vi "ParseAquatrakRange.vi"(8 "error in":errorcluster, 11 "Incoming String":string) -> (0 "error out":errorcluster, 1 "Cal Counts":i32, 2 "Valid Data":bool, 3 "Range":dbl, 5 "Range Counts":i32)   [LabVIEW 2019, in "Acquisition.lvlib"]
doc: "This VI takes an incoming string from the 4100 model Aquatrak controller and then outputs the quality as a Good Data = true/false boolean indicator."
uses:
  Acquisition/Acquisition.lvlib
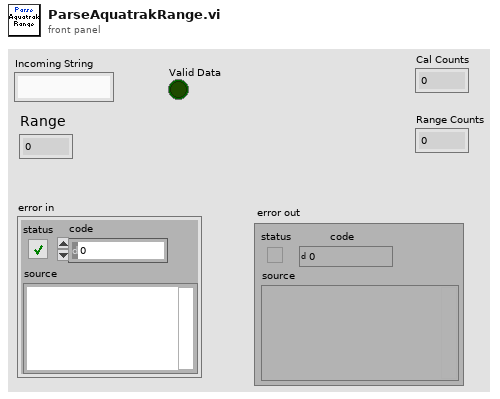
[diagram p1: front panel]
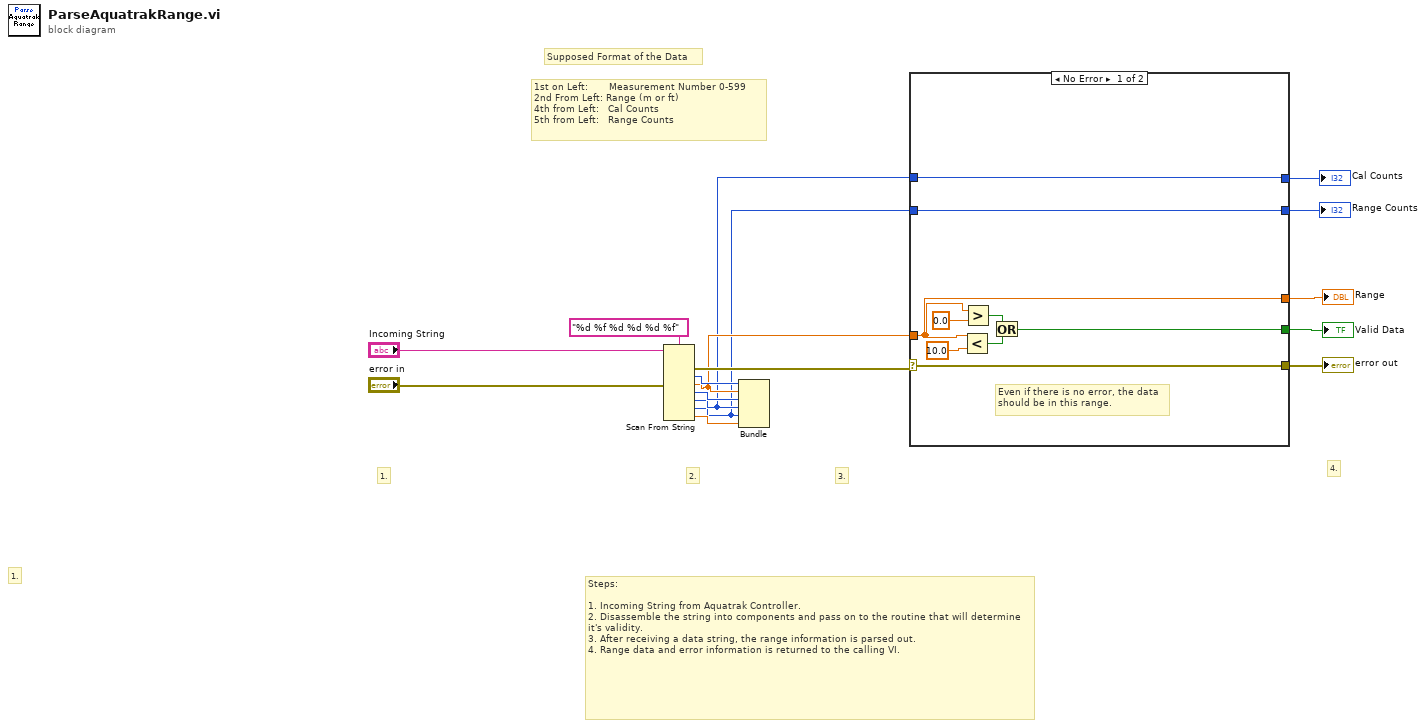
[diagram p0: block diagram]
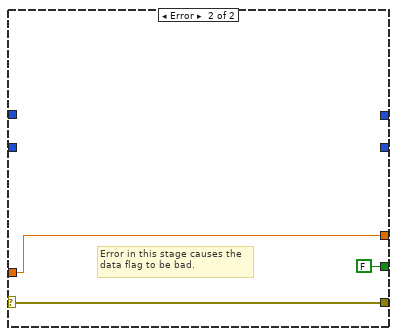
[diagram p2: hidden frame]
diagram:
  # "1st on Left:       Measurement Number 0-599\n2nd From Left: Range (m or ft)\n4th from Left:   Cal Counts\n5th from Left:   Range Counts"
  # "4."
  # "Supposed Format of the Data"
  # "Steps:\n\n1. Incoming String from Aquatrak Controller.\n2. Disassemble the string into components and pass on to the routine that will determine it's validity.\n3. After receiving a data string, the range information is parsed out.\n4. Range data and error information is returned to the calling VI."
  # "3."
  # "2."
  # "1."
  # "1."
  n1 = Scan From String(format string="%d %f %d %d %d %f", input string="Incoming String", error in="error in") -> (error out=w9:errorcluster, output 1=w13:i32, output 2=w7:dbl, output 3=w14:i32, output 4=w4:i32, output 5=w3:i32, output 6=w15:dbl)  [unwired: 7 in, 2 out]
  n2 = Bundle(w13, w7, w14, w4, w3, w15) -> ()  [unwired: 1 in, 1 out]
  n3 = case shown="No Error" w9 {
    selector: w9 -> [w24 w27]
    tunnel: [w24 w27] -> w8
    tunnel: w7 -> [w19 w25]
    tunnel: [w19 w25] -> w6
    tunnel: [w18 FALSE] -> w5
    tunnel: w4 -> [w17 _]
    tunnel: w3 -> [w16 _]
    tunnel: [w17 _] -> w2
    tunnel: [w16 _] -> w1
    frame No Error {
      # "Even if there is no error, the data\nshould be in this range."
      n4 = Less?(x=w19, y=10.0) -> (x < y?=w23:bool)
      n5 = Greater?(x=w19, y=0.0) -> (0:w22:bool)
      n6 = Or(x=w22, y=w23) -> (x .or. y?=w18:bool)
    }
    frame Error {
      # "Error in this stage causes the \ndata flag to be bad."
    }
  }
  "error out" <- w8
  "Range" <- w6
  "Valid Data" <- w5
  "Cal Counts" <- w2
  "Range Counts" <- w1
